vi "Gain Zee.vi"(5 "Sample Rate":dbl format="%.2f", 6 "Number of Impulses":i32, 7 "Graph Cluster":T1={"Plot Traces"=[{"Color Box"=4652800, "Boolean"=TRUE, "List 2"=5, "Boolean 2"=FALSE, "Boolean 3"=TRUE, "Offset"=0.0, "Gain"=1.0}, {"Color Box"=16733696, "Boolean"=TRUE, "List 2"=13, "Boolean 2"=TRUE, "Boolean 3"=TRUE, "Offset"=0.0, "Gain"=1.0}, {"Color Box"=393436, "Boolean"=TRUE, "List 2"=21, "Boolean 2"=TRUE, "Boolean 3"=TRUE, "Offset"=0.0, "Gain"=1.0}], "Gain Calculations"={"Threshold Trace"=0, "Min Thresh/%"=0.0, "Max Thresh/%"=0.0, "Gain calculated by dividing"=0, "Gain Range"=enum."Peak %", "Pre-peak-ms"=0.0, "by"=0}, "Impulse Plane"=enum."LARP", "Impulse Direction"=TRUE} {"Gain Calculations"."by" items=["Hx Position-in-Head", "Hy Position-in-Head", "Hz Position-in-Head", "Hx Velocity-in-Head", "Hy Velocity-in-Head", "Hz Velocity-in-Head", "Hl Velocity-in-Head", "Hr Velocity-in-Head", "Lx Position-in-Head", "Ly Position-in-Head", "Lz Position-in-Head", "Lx Velocity-in-Head", "Ly Velocity-in-Head", "Lz Velocity-in-Head", "Ll Velocity-in-Head", "Lr Velocity-in-Head", "Rx Position-in-Head", "Ry Position-in-Head", "Rz Position-in-Head", "Rx Velocity-in-Head", "Ry Velocity-in-Head", "Rz Velocity-in-Head", "Rl Velocity-in-Head", "Rr Velocity-in-Head", "Button", "Ascension X", "Ascension X Vel", "Ascension Y", "Ascension Y Vel", "Ascension Z", "Ascension Z Vel", " "]; "Gain Calculations"."Pre-peak-ms" format="%.2f"; "Gain Calculations"."Gain calculated by dividing" items=["Hx Position-in-Head", "Hy Position-in-Head", "Hz Position-in-Head", "Hx Velocity-in-Head", "Hy Velocity-in-Head", "Hz Velocity-in-Head", "Hl Velocity-in-Head", "Hr Velocity-in-Head", "Lx Position-in-Head", "Ly Position-in-Head", "Lz Position-in-Head", "Lx Velocity-in-Head", "Ly Velocity-in-Head", "Lz Velocity-in-Head", "Ll Velocity-in-Head", "Lr Velocity-in-Head", "Rx Position-in-Head", "Ry Position-in-Head", "Rz Position-in-Head", "Rx Velocity-in-Head", "Ry Velocity-in-Head", "Rz Velocity-in-Head", "Rl Velocity-in-Head", "Rr Velocity-in-Head", "Button", "Ascension X", "Ascension X Vel", "Ascension Y", "Ascension Y Vel", "Ascension Z", "Ascension Z Vel", " "]; "Gain Calculations"."Max Thresh/%" format="%.2f"; "Gain Calculations"."Min Thresh/%" format="%.2f"; "Gain Calculations"."Threshold Trace" items=["Hx Position-in-Head", "Hy Position-in-Head", "Hz Position-in-Head", "Hx Velocity-in-Head", "Hy Velocity-in-Head", "Hz Velocity-in-Head", "Hl Velocity-in-Head", "Hr Velocity-in-Head", "Lx Position-in-Head", "Ly Position-in-Head", "Lz Position-in-Head", "Lx Velocity-in-Head", "Ly Velocity-in-Head", "Lz Velocity-in-Head", "Ll Velocity-in-Head", "Lr Velocity-in-Head", "Rx Position-in-Head", "Ry Position-in-Head", "Rz Position-in-Head", "Rx Velocity-in-Head", "Ry Velocity-in-Head", "Rz Velocity-in-Head", "Rl Velocity-in-Head", "Rr Velocity-in-Head", "Button", "Ascension X", "Ascension X Vel", "Ascension Y", "Ascension Y Vel", "Ascension Z", "Ascension Z Vel", " "]; "Plot Traces"."Gain" format="%.1f"; "Plot Traces"."Offset" format="%.1f"; "Plot Traces"."List 2" items=["Hx Position-in-Head", "Hy Position-in-Head", "Hz Position-in-Head", "Hx Velocity-in-Head", "Hy Velocity-in-Head", "Hz Velocity-in-Head", "Hl Velocity-in-Head", "Hr Velocity-in-Head", "Lx Position-in-Head", "Ly Position-in-Head", "Lz Position-in-Head", "Lx Velocity-in-Head", "Ly Velocity-in-Head", "Lz Velocity-in-Head", "Ll Velocity-in-Head", "Lr Velocity-in-Head", "Rx Position-in-Head", "Ry Position-in-Head", "Rz Position-in-Head", "Rx Velocity-in-Head", "Ry Velocity-in-Head", "Rz Velocity-in-Head", "Rl Velocity-in-Head", "Rr Velocity-in-Head", "Button", "Ascension X", "Ascension X Vel", "Ascension Y", "Ascension Y Vel", "Ascension Z", "Ascension Z Vel", " "]}, 9 "Data (in)":dbl[][](array[numeric]) format="%.2f") -> (0 "STD":dbl format="%.2f", 1 "STD array":dbl[](array[numeric]) format="%.2f", 3 "GAIN":dbl format="%.2f")   [LabVIEW 2016, in "generate report.lvlib"]
uses:
  generate report.lvlib
  <vilib>/Analysis/baseanly.llb/Mean (DBL).vi
  comm/stats/stats.lvlib
  <vilib>/Analysis/NI_AALBase.lvlib
panel:
  # "Copyright Americo A. Migliaccio (c) 2002 All Rights Reserved by Author"
  # "-"
  # "+"
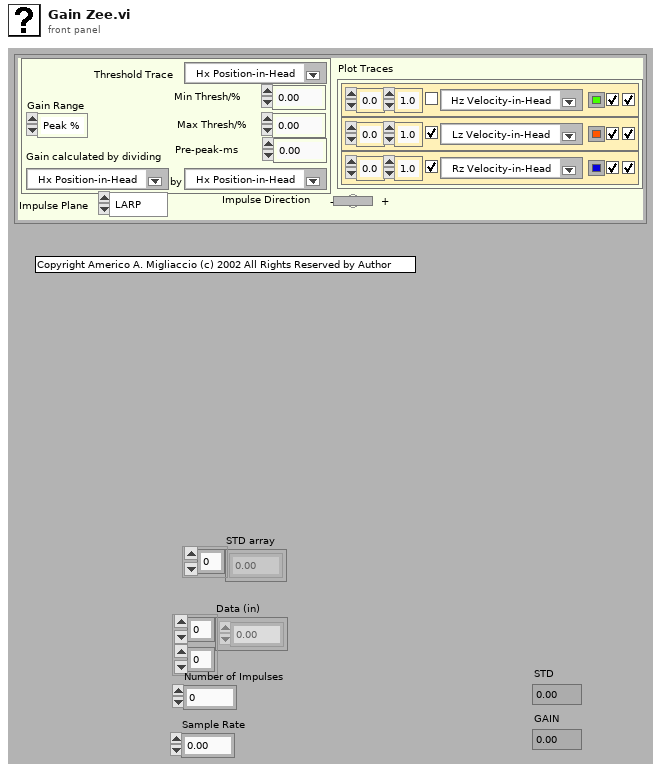
[diagram p1: front panel]
types:
  T1 = cluster{"Plot Traces":cluster{"Color Box":u32, "Boolean":bool, "List 2":u16, "Boolean 2":bool, "Boolean 3":bool, "Offset":dbl, "Gain":dbl}[], "Gain Calculations":cluster{"Threshold Trace":u16, "Min Thresh/%":dbl, "Max Thresh/%":dbl, "Gain calculated by dividing":u16, "Gain Range":enum16{"Peak %", "Best Est", "Thresh"}, "Pre-peak-ms":dbl, "by":u16}, "Impulse Plane":enum16{"Other", "Yaw", "Pitch", "Roll", "LARP", "RALP"}, "Impulse Direction":bool}
  T2 = cluster{"Color Box":u32, "Boolean":bool, "List 2":u16, "Boolean 2":bool, "Boolean 3":bool, "Offset":dbl, "Gain":dbl}[]
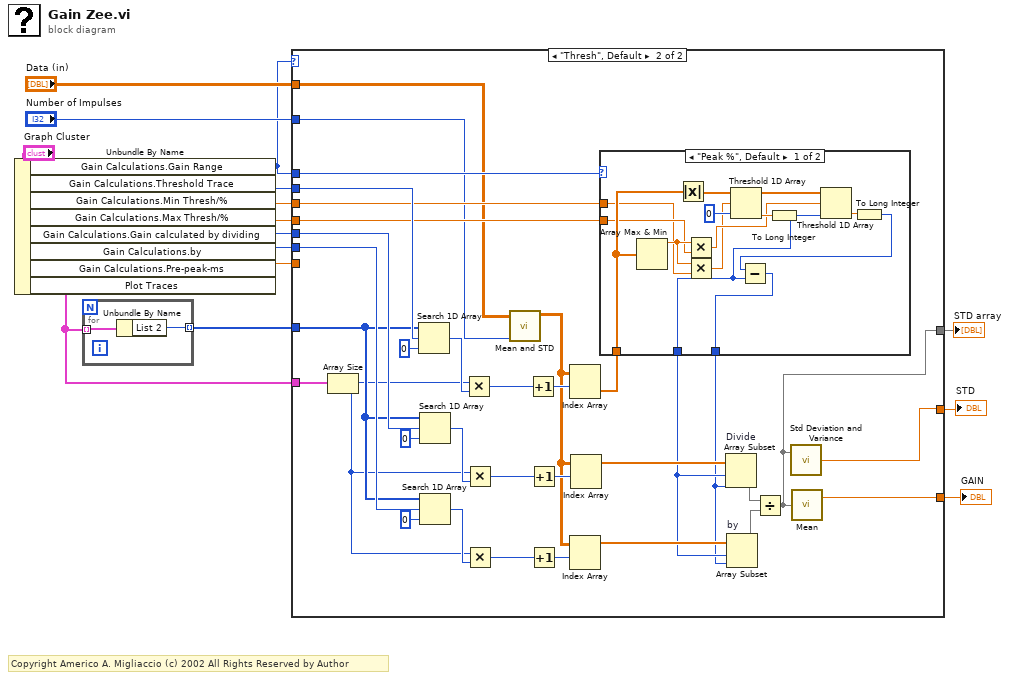
[diagram p0: block diagram]
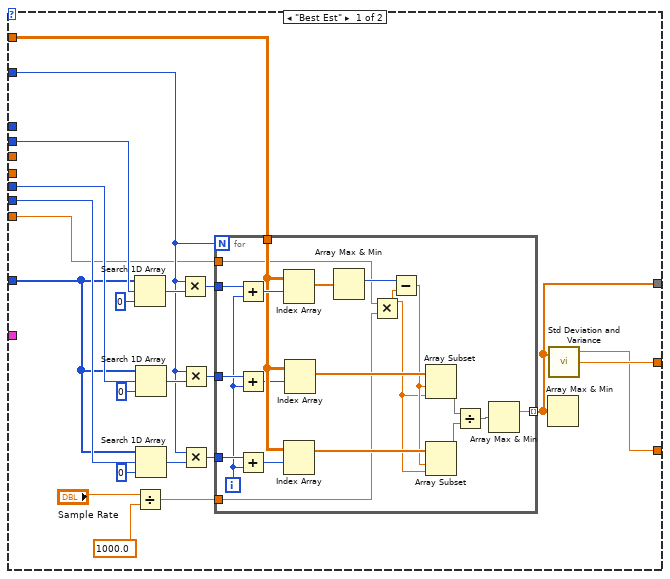
[diagram p2: hidden frame]
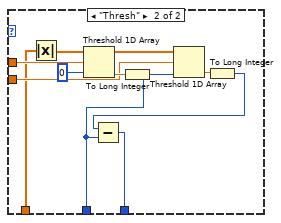
[diagram p3: hidden frame]
diagram:
  # "Copyright Americo A. Migliaccio (c) 2002 All Rights Reserved by Author"
  n1 = Unbundle By Name("Graph Cluster") -> ("Gain Calculations.Gain Range"=w6:enum16{"Peak %", "Best Est", "Thresh"}, "Gain Calculations.Threshold Trace"=w15:u16, "Gain Calculations.Min Thresh/%"=w12:dbl, "Gain Calculations.Max Thresh/%"=w11:dbl, "Gain Calculations.Gain calculated by dividing"=w14:u16, "Gain Calculations.by"=w13:u16, "Gain Calculations.Pre-peak-ms"=w5:dbl, "Plot Traces"=w4:T2)
  n2 = for {
    tunnel: w4 -> [w17] mode=indexing
    tunnel: [w16] -> w8 mode=indexing
    n3 = Unbundle By Name(w17) -> ("List 2"=w16:u16)
  }
  n4 = case shown="\"Thresh\", Default" w6 {
    tunnel: w15 -> [w29 w93]
    tunnel: w14 -> [w28 w92]
    tunnel: w13 -> [w27 w91]
    tunnel: w12 -> [_ w90]
    tunnel: w11 -> [_ w89]
    tunnel: w6 -> [_ w88]
    tunnel: "Data (in)" -> [w30 w87]
    tunnel: "Number of Impulses" -> [w25 w86]
    tunnel: w8 -> [w26 w79]
    tunnel: w4 -> [_ w64]
    tunnel: [w19 w62] -> w7
    tunnel: w5 -> [w24 _]
    tunnel: [w20 w61] -> w2
    tunnel: [w18 w60] -> w1
    frame "Best Est" {
      n5 = Search 1D Array(1D array=w26, element=w29, start index (0)=0) -> (index of element=w38:i32)
      n6 = Divide(x="Sample Rate", y=1000.0) -> (x/y=w21:dbl)
      n7 = Search 1D Array(1D array=w26, element=w28, start index (0)=0) -> (index of element=w37:i32)
      n8 = Search 1D Array(1D array=w26, element=w27, start index (0)=0) -> (index of element=w34:i32)
      n9 = Multiply(x=w25, y=w38) -> (x*y=w33:i32)
      n10 = Multiply(x=w25, y=w37) -> (x*y=w32:i32)
      n11 = Multiply(x=w25, y=w34) -> (x*y=w31:i32)
      n12 = for {
        N: w25 -> [_]
        tunnel: w30 -> [w55]
        tunnel: w33 -> [w57]
        tunnel: w32 -> [w59]
        tunnel: w31 -> [w58]
        tunnel: [w40] -> w18 mode=indexing
        tunnel: w24 -> [w44]
        tunnel: w21 -> [w43]
        i -> [w52]
        n13 = Add(x=w57, y=w52) -> (x+y=w56:i32)
        n14 = Add(x=w59, y=w52) -> (x+y=w54:i32)
        n15 = Add(x=w58, y=w52) -> (x+y=w53:i32)
        n16 = Index Array(array=w55, index (row)=w56) -> (element=w51:dbl[])  [unwired: 1 in]
        n17 = Index Array(array=w55, index (row)=w53) -> (element=w48:dbl[])  [unwired: 1 in]
        n18 = Index Array(array=w55, index (row)=w54) -> (element=w49:dbl[])  [unwired: 1 in]
        n19 = Array Max & Min(array=w51) -> (max index (indices)=w50:i32)  [unwired: 3 out]
        n20 = Multiply(x=w44, y=w43) -> (x*y=w42:dbl)
        n21 = Subtract(x=w50, y=w42) -> (x-y=w47:dbl)
        n22 = Array Subset(array=w49, index=w47, length=w42) -> (w46:dbl[])
        n23 = Array Subset(array=w48, index=w47, length=w42) -> (w45:dbl[])
        n24 = Divide(x=w46, y=w45) -> (x/y=w41:dbl[])
        n25 = Array Max & Min(array=w41) -> (max value=w40:dbl)  [unwired: 3 out]
      }
      n26 = Array Max & Min(array=w18) -> ()  [unwired: 4 out]
      n27 = call "Std Deviation and Variance.vi"("X"=w18) -> ("mean"=w19:dbl, "standard deviation"=w20:dbl)  [unwired: 1 in, 1 out]
    }
    frame "Thresh", Default {
      n28 = Array Size(array=w64) -> (size(s)=w63:i32)
      n29 = Search 1D Array(1D array=w79, element=w93, start index (0)=0) -> (index of element=w83:i32)
      n30 = Search 1D Array(1D array=w79, element=w92, start index (0)=0) -> (index of element=w82:i32)
      n31 = Search 1D Array(1D array=w79, element=w91, start index (0)=0) -> (index of element=w76:i32)
      n32 = Multiply(x=w63, y=w83) -> (x*y=w85:i32)
      n33 = Multiply(x=w63, y=w82) -> (x*y=w80:i32)
      n34 = Multiply(x=w63, y=w76) -> (x*y=w78:i32)
      n35 = call "Mean and STD.vi"("Data (in)"=w87, "Number of Impulses"=w86) -> ("Mean and STD"=w65:dbl[][])  [unwired: 11 in, 2 out]
      n36 = Increment(x=w85) -> (x+1=w75:i32)
      n37 = Increment(x=w80) -> (x+1=w74:i32)
      n38 = Increment(x=w78) -> (x+1=w73:i32)
      n39 = Index Array(array=w65, index (row)=w75) -> (element=w72:dbl[])  [unwired: 1 in]
      n40 = Index Array(array=w65, index (row)=w73) -> (element=w70:dbl[])  [unwired: 1 in]
      n41 = Index Array(array=w65, index (row)=w74) -> (element=w71:dbl[])  [unwired: 1 in]
      n42 = case shown="\"Peak %\", Default" w88 {
        tunnel: w90 -> [w94 w111]
        tunnel: w89 -> [w95 w110]
        tunnel: w72 -> [w99 w109]
        tunnel: [w101 w108] -> w69
        tunnel: [w100 w107] -> w68
        frame "Peak %", Default {
          n43 = Array Max & Min(array=w99) -> (max value=w98:dbl)  [unwired: 3 out]
          n44 = Absolute Value(x=w99) -> (abs(x)=w106:dbl[])
          n45 = Multiply(x=w98, y=w95) -> (x*y=w97:dbl)
          n46 = Multiply(x=w98, y=w94) -> (x*y=w96:dbl)
          n47 = Threshold 1D Array(1:0 ("start index (0)"), 2:w96, 3:w106) -> (0:w102:dbl)
          n48 = To Long Integer(number=w102) -> (32bit integer=w101:i32)
          n49 = Threshold 1D Array(1:w101, 2:w97, 3:w106) -> (0:w103:dbl)
          n50 = To Long Integer(number=w103) -> (32bit integer=w104:i32)
          n51 = Subtract(x=w104, y=w101) -> (x-y=w100:i32)
        }
        frame "Thresh" {
          n52 = Absolute Value(x=w109) -> (abs(x)=w116:dbl[])
          n53 = Threshold 1D Array(1:0 ("start index (0)"), 2:w111, 3:w116) -> (0:w112:dbl)
          n54 = To Long Integer(number=w112) -> (32bit integer=w108:i32)
          n55 = Threshold 1D Array(1:w108, 2:w110, 3:w116) -> (0:w113:dbl)
          n56 = To Long Integer(number=w113) -> (32bit integer=w114:i32)
          n57 = Subtract(x=w114, y=w108) -> (x-y=w107:i32)
        }
      }
      n58 = Array Subset "Divide"(array=w71, index=w69, length=w68) -> (w67:dbl[])
      n59 = Array Subset "by"(array=w70, index=w69, length=w68) -> (w66:dbl[])
      n60 = Divide(x=w67, y=w66) -> (x/y=w60:dbl[])
      n61 = call "Std Deviation and Variance.vi"("X"=w60) -> ("standard deviation"=w61:dbl)  [unwired: 1 in, 2 out]
      n62 = call-poly <vilib>:"Mean.vi"("X"=w60) -> ("mean"=w62:dbl)  [unwired: 1 out]
    }
  }
  "GAIN" <- w7
  "STD" <- w2
  "STD array" <- w1
